vi "Horizontal Next Sample Rate.vi"(8 "error in":errorcluster, 9 "steps":i32(ring) caption="Increment Type" items=["ZTSCOPEM_INCREMENT", "ZTSCOPEM_DECREMENT"], 10 "Sample Rate In":dbl, 11 "Instrument Handle In":i32) -> (0 "error out":errorcluster, 1 "Next Rate":dbl, 2 "Sample Rate Out":dbl, 3 "Instrument Handle Out":i32)   [LabVIEW 8.6, in "ZTScopeM.lvlib"]
doc: "Query what the sample rate is, based on the passed in Sample Rate and Increment Type."
uses:
  ZTScopeM.lvlib
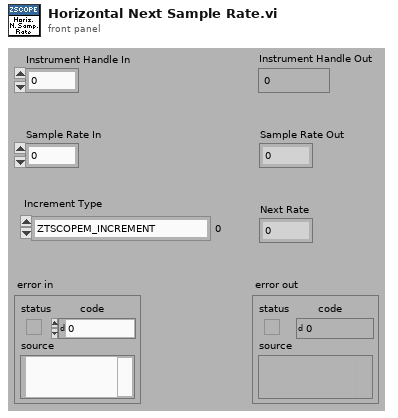
[diagram p1: front panel]
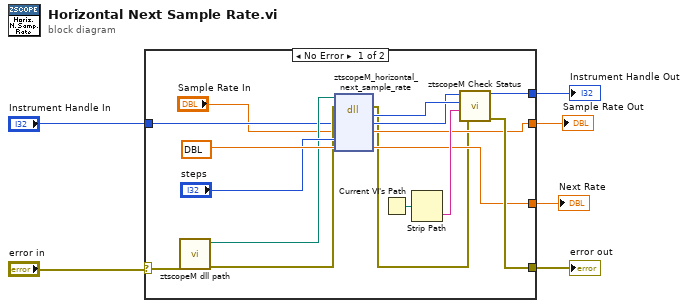
[diagram p0: block diagram]
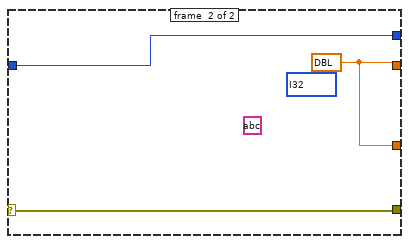
[diagram p2: hidden frame]
diagram:
  n1 = case shown="No Error" "error in" {
    selector: "error in" -> [w12 w25]
    tunnel: [w17 w25] -> w5
    tunnel: [w18 w23] -> w4
    tunnel: [w16 w24] -> w3
    tunnel: [w15 w24] -> w2
    tunnel: "Instrument Handle In" -> [w8 w23]
    frame #0 {
      n2 = call "ztscopeM dll path.vi"("error in (no error)"=w12) -> ("error out"=w10:errorcluster, "<instrument>.dll path"=w11:path)  [unwired: 9 in]
      n3 = dll-call lib="C:/Program Files (x86)/National Instruments/LabVIEW 2013/instr.lib/ztscopem/ztscopeM.dll" fn="ztscopeM_horizontal_next_sample_rate"(path in=w11, error in=w10, "instrumentHandle"=w8, "sampleRate"="Sample Rate In", "incrementType"="steps", "nextRate"=dbl ? ("sampleRate")) -> (error out=w9:errorcluster, "return type"=w22:i32, "instrumentHandle"=w21:i32, "sampleRate"=w15:dbl, "nextRate"=w16:dbl)  [unwired: 1 in, 2 out]
      n4 = Current VI's Path() -> (path=w20:path)
      n5 = Strip Path(path=w20) -> (name=w19:string)  [unwired: 1 out]
      n6 = call "ztscopeM Check Status.vi"("error in"=w9, "name of VI"=w19, "status (return code)"=w22, "instrument handle in"=w21) -> ("error out"=w17:errorcluster, "instrument handle out"=w18:i32)  [unwired: 2 out]
    }
    frame #1 {
      w24 = dbl ? ("sampleRate")
      (unwired) i32[] ? ("incrementType")
      (unwired) string ? ("driverRev")
    }
  }
  "Instrument Handle Out" <- w4
  "error out" <- w5
  "Next Rate" <- w3
  "Sample Rate Out" <- w2
